vi "intNegate.vi"(8 "Error in (no error)":errorcluster, 11 "Int in":refnum<class "IntClass.lvclass">) -> (0 "Error out":errorcluster, 3 "Int out":refnum<class "IntClass.lvclass">)   [LabVIEW 2011, in "IntClass.lvclass"]
uses:
  IntClass.lvclass
  IntClass.lvclass/IntClass.ctl
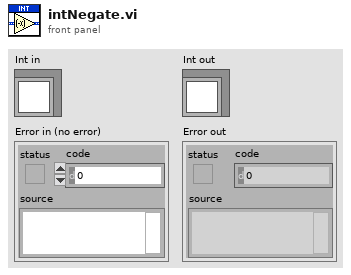
[diagram p1: front panel]
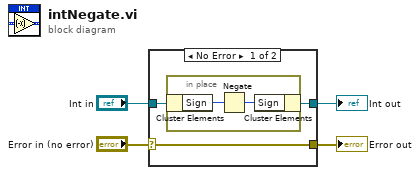
[diagram p0: block diagram]
diagram:
  n1 = case shown="No Error" "Error in (no error)" {
    selector: "Error in (no error)" -> [w7 w10]
    tunnel: [w7 w10] -> w3
    tunnel: "Int in" -> [w6 _]
    tunnel: [w5 _] -> w1
    frame No Error {
      n2 = in-place {
        n3 = in-place-cluster #1(w6) -> ("Sign"=w9:i8)
        n4 = Negate(x=w9) -> (-x=w8:i8)
        n5 = in-place-cluster #1("Sign"=w8) -> (w5:refnum<class "IntClass.lvclass">)
      }
    }
    frame Error {
    }
  }
  "Int out" <- w1
  "Error out" <- w3
